vi "CreateServer.vi"() -> (3 "gRPCid":T1)   [LabVIEW 2019, in "gprc-support.lvlib"]
uses:
  gprc-support.lvlib
  grpcId.ctl
  build/Debug/labview_grpc_server.dll
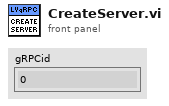
[diagram p1: front panel]
types:
  T1 = typedef "gprc-support.lvlib/grpcId.ctl" = u64
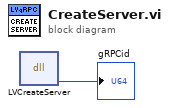
[diagram p0: block diagram]
diagram:
  n1 = dll-call lib="C:/dev/labview-grpc-server/build/Debug/labview_grpc_server.dll" fn="LVCreateServer"() -> ("gRPCid"=→"gRPCid":T1)  [unwired: 5 in, 2 out]
